vi "Sample Report (Word).vi"() -> ()   [LabVIEW 2020]
doc: "This example shows how to use high-level Word Specific VIs to generate a test report."
uses:
  <vilib>/addons/_office/word.llb/Word Easy Table (str).vi
  <vilib>/Utility/NIReport.llb/NI_report.lvclass
  <vilib>/addons/_office/NI_ReportGenerationToolkit.lvlib
  <vilib>/Utility/NIReport.llb/Word/NI_Word.lvclass
panel:
  in  "Text":string="Description: This example shows how to use high-level Word Specific VIs to generate a test report.\n\n\n\n\n"
  in  "Table":string[][](table)=[["1", "1.5", "5.6", "5.6", "7.9", "4.6"], ["2", "2.5", "7.6", "6.5", "7.2", "7.5"], ["3", "6.8", "9.1", "4.2", "6.2", "6.1"], ["4", "6.7", "7.1", "7.2", "1.0", "8.3"], ["5", "6.4", "4.3", "9.2", "5.8", "4.2"], ["6", "8.6", "8.2", "4.3", "8.6", "4.5"]]
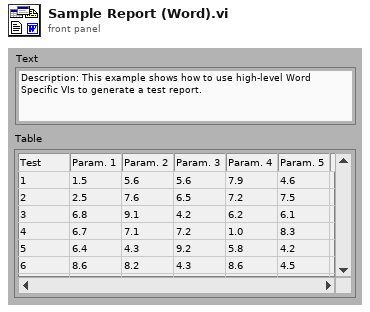
[diagram p1: front panel]
types:
  T1 = enum16{"wdLineStyleNone", "wdLineStyleSingle", "wdLineStyleDot", "wdLineStyleDashSmallGap", "wdLineStyleDashLargeGap", "wdLineStyleDashDot", "wdLineStyleDashDotDot", "wdLineStyleDouble", "wdLineStyleTriple", "wdLineStyleThinThickSmallGap", "wdLineStyleThickThinSmallGap", "wdLineStyleThinThickThinSmallGap", "wdLineStyleThinThickMedGap", "wdLineStyleThickThinMedGap", "wdLineStyleThinThickThinMedGap", "wdLineStyleThinThickLargeGap", "wdLineStyleThickThinLargeGap", "wdLineStyleThinThickThinLargeGap", "wdLineStyleSingleWavy", "wdLineStyleDoubleWavy", "wdLineStyleDashDotStroked", "wdLineStyleEmboss3D", "wdLineStyleEngrave3D", "wdLineStyleOutset", "wdLineStyleInset"}
  T2 = enum16{"Standard Report", "HTML", "Word", "Excel"}
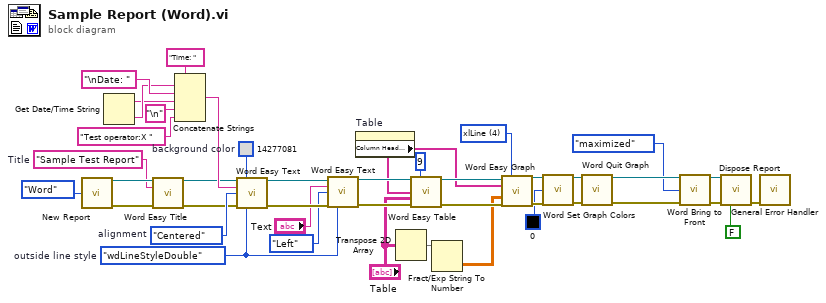
[diagram p0: block diagram]
diagram:
  w23 = "Sample Test Report"  # Title
  w13 = u32 14277081  # background color
  w18 = 4 items=["xlColumnClustered"=51, "xlColumnStacked"=52, "xlColumnStacked100"=53, "xl3DColumnClustered"=54, "xl3DColumnStacked"=55, "xl3DColumnStacked100"=56, "xlBarClustered"=57, "xlBarStacked"=58, "xlBarStacked100"=59, "xl3DBarClustered"=60, "xl3DBarStacked"=61, "xl3DBarStacked100"=62, "xlLineStacked"=63, "xlLineStacked100"=64, "xlLineMarkers"=65, "xlLineMarkersStacked"=66, "xlLineMarkersStacked100"=67, "xlPieOfPie"=68, "xlPieExploded"=69, "xl3DPieExploded"=70, "xlBarOfPie"=71, "xlXYScatterSmooth"=72, "xlXYScatterSmoothNoMarkers"=73, "xlXYScatterLines"=74, "xlXYScatterLinesNoMarkers"=75, "xlAreaStacked"=76, "xlAreaStacked100"=77, "xl3DAreaStacked"=78, "xl3DAreaStacked100"=79, "xlDoughnutExploded"=80, "xlRadarMarkers"=81, "xlRadarFilled"=82, "xlSurface"=83, "xlSurfaceWireframe"=84, "xlSurfaceTopView"=85, "xlSurfaceTopViewWireframe"=86, "xlBubble"=15, "xlBubble3DEffect"=87, "xlStockHLC"=88, "xlStockOHLC"=89, "xlStockVHLC"=90, "xlStockVOHLC"=91, "xlCylinderColClustered"=92, "xlCylinderColStacked"=93, "xlCylinderColStacked100"=94, "xlCylinderBarClustered"=95, "xlCylinderBarStacked"=96, "xlCylinderBarStacked100"=97, "xlCylinderCol"=98, "xlConeColClustered"=99, "xlConeColStacked"=100, "xlConeColStacked100"=101, "xlConeBarClustered"=102, "xlConeBarStacked"=103, "xlConeBarStacked100"=104, "xlConeCol"=105, "xlPyramidColClustered"=106, "xlPyramidColStacked"=107, "xlPyramidColStacked100"=108, "xlPyramidBarClustered"=109, "xlPyramidBarStacked"=110, "xlPyramidBarStacked100"=111, "xlPyramidCol"=112, "xl3DColumn"=-4100, "xlLine"=4, "xl3DLine"=-4101, "xl3DPie"=-4102, "xlPie"=5, "xlXYScatter"=-4169, "xl3DArea"=-4098, "xlArea"=1, "xlDoughnut"=-4120, "xlRadar"=-4151] ("chart type")
  w29 = enum16{"Left", "Centered", "Right", "Justify"}."Centered"  # alignment
  w31 = T1."wdLineStyleDouble"  # outside line style
  n1 = call <vilib>:"New Report.vi"("report type"=T2."Word") -> ("report out"=w25:refnum<class "NI_report.lvclass">, "error out"=w27:errorcluster)  [unwired: 13 in]
  n2 = Get Date/Time String() -> (date string=w5:string, time string=w6:string)  [unwired: 3 in]
  n3 = call <vilib>:"Word Easy Title.vi"("report in"=w25, "title"=w23, "error in (no error)"=w27) -> ("report out"=w24:refnum<class "NI_report.lvclass">, "error out"=w26:errorcluster)  [unwired: 10 in, 1 out]
  n4 = Concatenate Strings("Time: " ("Substring"), w6, "\nDate: " ("Substring"), w5, "\n" ("Substring"), "Test operator:X " ("Substring")) -> (w37:string)
  n5 = call <vilib>:"Word Easy Text.vi"("report in"=w24, "background pattern color (w)"=w13, "text"=w37, "alignment (left)"=w29, "error in (no error)"=w26, "outside line style (none)"=w31) -> ("report out"=w34:refnum<class "NI_report.lvclass">, "error out"=w35:errorcluster)  [unwired: 7 in, 1 out]
  n6 = call <vilib>:"Word Easy Text.vi"("report in"=w34, "text"="Text", "alignment (left)"=enum16{"Left", "Centered", "Right", "Justify"}."Left" ("alignment"), "error in (no error)"=w35, "outside line style (none)"=w31) -> ("report out"=w32:refnum<class "NI_report.lvclass">, "error out"=w33:errorcluster)  [unwired: 8 in, 1 out]
  n7 = property on="Table" class="Tbl (strict)"() -> ("Column Header Strings[]"=w17:string[])  [unwired: 2 in, 2 out]
  n8 = Transpose 2D Array(2D array="Table") -> (transposed array=w16:string[][])
  n9 = call-poly <vilib>:"Word Easy Table.vi"("report in"=w32, "auto format (none)"=9 ("autoformat"), "column headers"=w17, "data"="Table", "error in (no error)"=w33) -> ("report out"=w21:refnum<class "NI_report.lvclass">, "error out"=w22:errorcluster)  [unwired: 8 in, 1 out]
  n10 = Fract/Exp String To Number(string=w16) -> (number=w19:dbl[][])  [unwired: 3 in, 1 out]
  n11 = call <vilib>:"Word Easy Graph.vi"("report in"=w21, "graph type (col clustered)"=w18, "row headers"=w17, "data"=w19, "error in (no error)"=w22) -> ("report out"=w14:refnum<class "NI_report.lvclass">, "error out"=w15:errorcluster)  [unwired: 9 in]
  n12 = call <vilib>:"Word Set Graph Colors.vi"("report in"=w14, "graph area color (w)"=u32 0 ("plot area color"), "error in (no error)"=w15) -> ("report out"=w10:refnum<class "NI_report.lvclass">, "error out"=w11:errorcluster)  [unwired: 11 in]
  n13 = call <vilib>:"Word Quit Graph.vi"("report in"=w10, "error in (no error)"=w11) -> ("report out"=w8:refnum<class "NI_report.lvclass">, "error out"=w9:errorcluster)  [unwired: 12 in]
  n14 = call <vilib>:"Word Bring to Front.vi"("report in"=w8, "window state (maximized)"=enum16{"maximized", "minimized", "normal"}."maximized", "error in (no error)"=w9) -> ("report out"=w3:refnum<class "NI_report.lvclass">, "error out"=w4:errorcluster)  [unwired: 11 in]
  n15 = call-dynamic "Dispose Report.vi"("report in"=w3, "error in (no error)"=w4, "close report? (T)"=FALSE ("Close Report? (T)")) -> ("error out"=w2:errorcluster)  [unwired: 12 in]
  n16 = call <vilib>:"General Error Handler.vi"("error in (no error)"=w2) -> ()  [unwired: 10 in, 5 out]
